vi "Actor Core.vi"(8 "error in":errorcluster, 11 "SLM_Controller in":refnum<class "SLM_Controller.lvclass">) -> (0 "error out":errorcluster, 3 "Actor out":refnum<class "Actor.lvclass">)   [LabVIEW 2023, in "SLM_Controller.lvlib" / "SLM_Controller.lvclass"]
doc: "(<B>Filename</B>: Actor Framework.lvlib:Actor.lvclass:Actor Core.vi)\n\nReceives messages to the actor, reacts to them, and initiates any error handling that may shut the actor down.\n\nDescendant classes may override this VI to append parallel tasks for the actor to complete while it handles messages. Overrides use the Call Parent Class Method node."
uses:
  SLM_Controller.lvclass
  C:/Program Files/National Instruments/LabVIEW 2023/vi.lib/ActorFramework/Actor/Actor.lvclass
  <vilib>/ActorFramework/Actor/Actor.lvclass
  <vilib>/ActorFramework/Actor/Actor.lvclass/Actor.ctl
  <vilib>/ActorFramework/Message Enqueuer/Message Enqueuer.lvclass/Message Enqueuer.ctl
  <vilib>/ActorFramework/Message Enqueuer/Init from Existing Queue.vi
  <vilib>/ActorFramework/Message Enqueuer/Enqueue.vi
  <vilib>/ActorFramework/Stop Msg/Stop Msg.lvclass
  C:/Program Files/National Instruments/LabVIEW 2023/vi.lib/ActorFramework/Message/Message.lvclass
  <vilib>/ActorFramework/Message Priority Queue/Priority Enqueue.vi
  <vilib>/ActorFramework/Message Enqueuer/Message Enqueuer.lvclass
  SLM_Controller.lvclass/SLM_Controller.ctl
panel:
  out "Main Control Path":path
  out "function name out":errorcluster
  out "Python Session":refnum<k35>
  out "Python Scripts Path":path
  out "VI":refnum<vi>
  out "Phase Array Graph":dbl[][](graph)
  in  "Continuous Button":bool
  in  "Correction Pattern":path=path "C:/Users/quantum/Documents/LVDAQ/ConcreteClasses/ConcreteInstrumentClasses/SLMClasses/Hamamatsu_X13138/Resources/correction_pattern_13138/CAL_LSH0802650_810nm.bmp"
  in  "SLM Monitor":i32=2
  in  "Modulation Depth":dbl=214.0
  in  "Initialize SLM":bool
  in  "Grating Sliders":cluster{"Y":sgl, "X":sgl} {"X" min=0 max=10 step=0.01 scale=0.0..10.0; "Y" min=0 max=10 step=0.01 scale=0.0..10.0}
  out "SLM Final Phase":dbl[][](graph)
  in  "Single Upload":bool
  in  "SLM Size":i32=800
  in  "Phase Array":dbl[][](array[numeric])
  in  "MegaPixels Y":i32=4
  in  "MegaPixels X":i32=4
  in  "Start/Stop":bool
  in  "Phase Scan ON / OFF":bool
  in  "Phase Scan":u16(ring) items=["2x1", "1x2", "2x2"]
  # "X"
  # "Y"
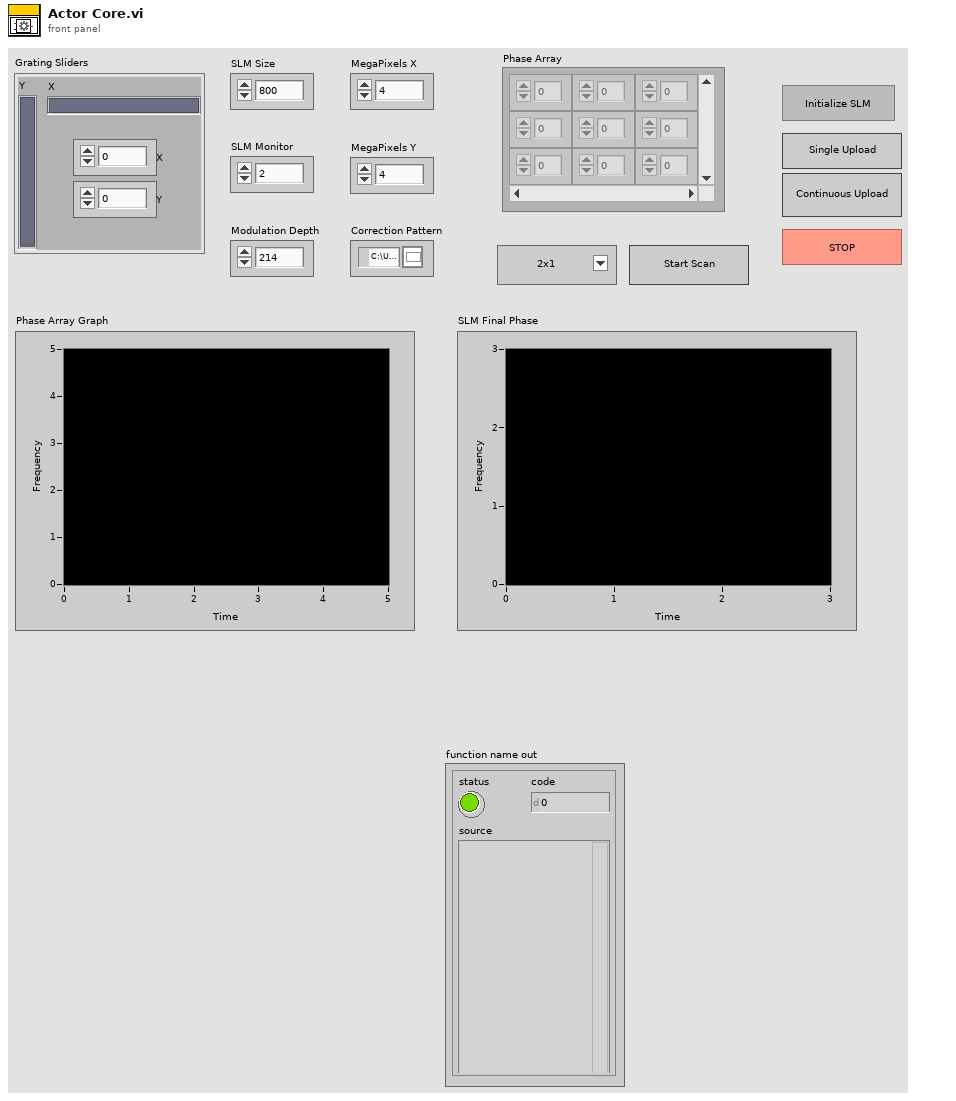
[diagram p1: front panel]
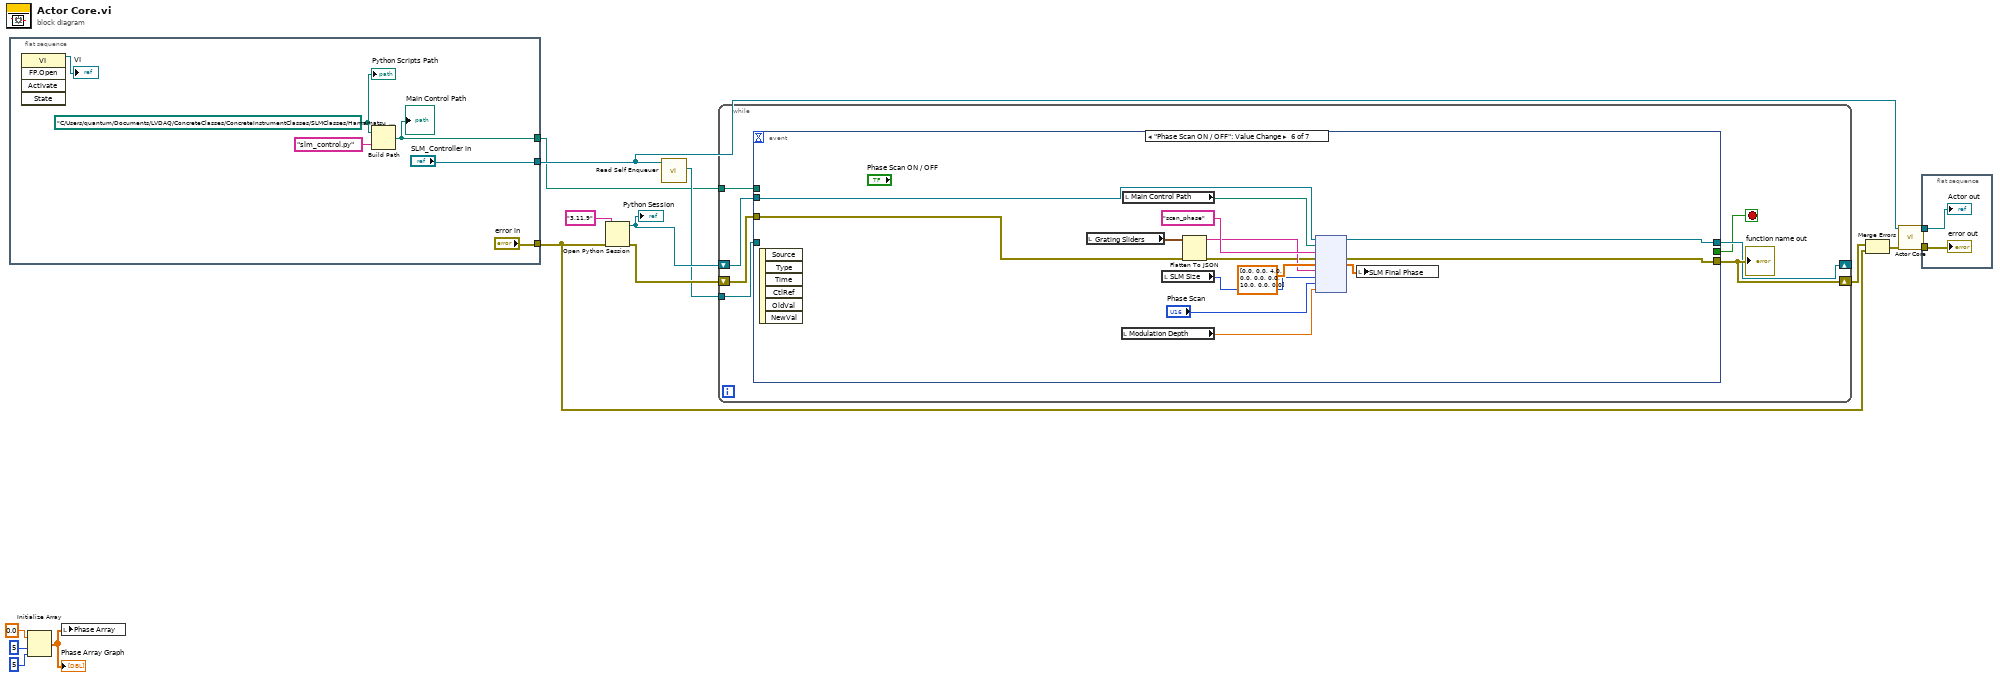
[diagram p0: block diagram]
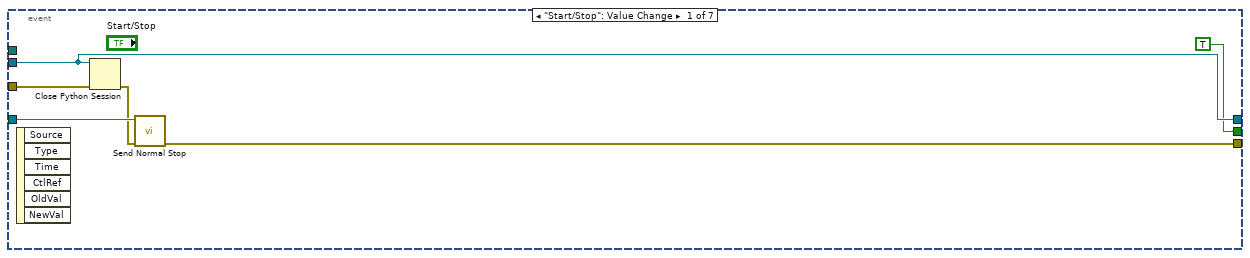
[diagram p2: hidden frame]
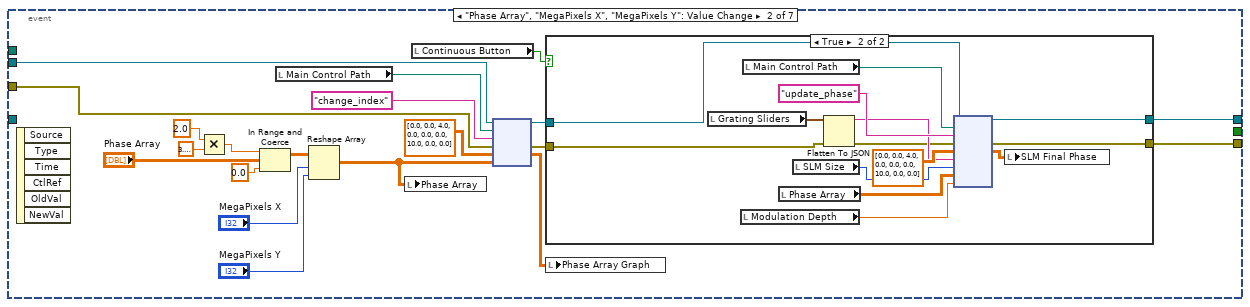
[diagram p3: hidden frame]
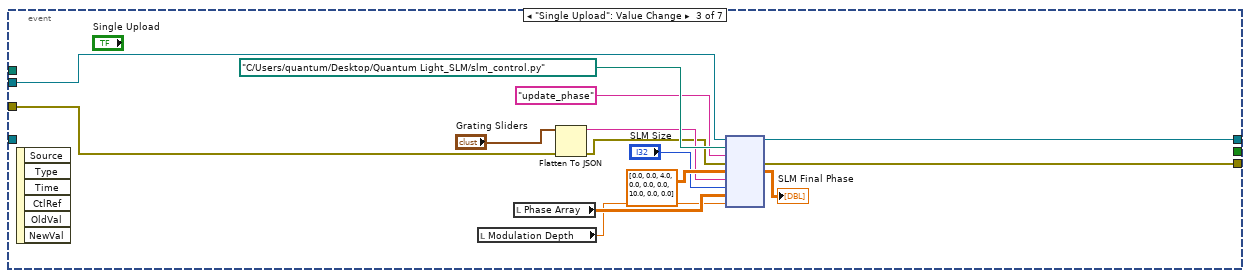
[diagram p5: hidden frame]
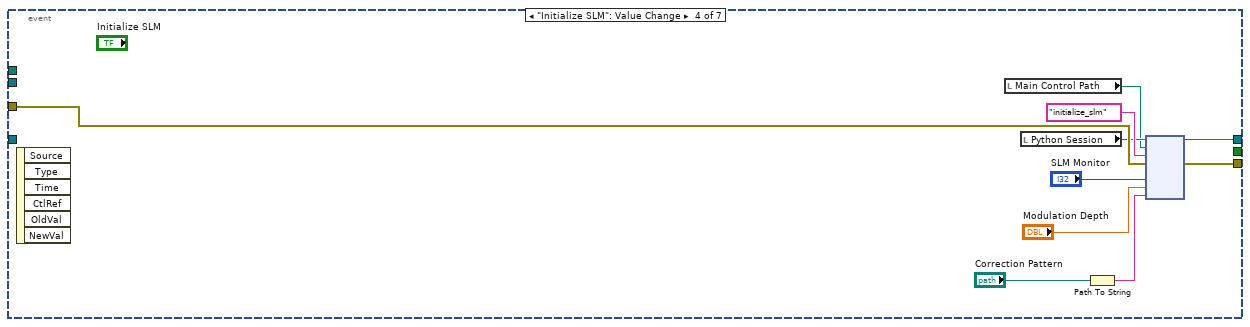
[diagram p6: hidden frame]
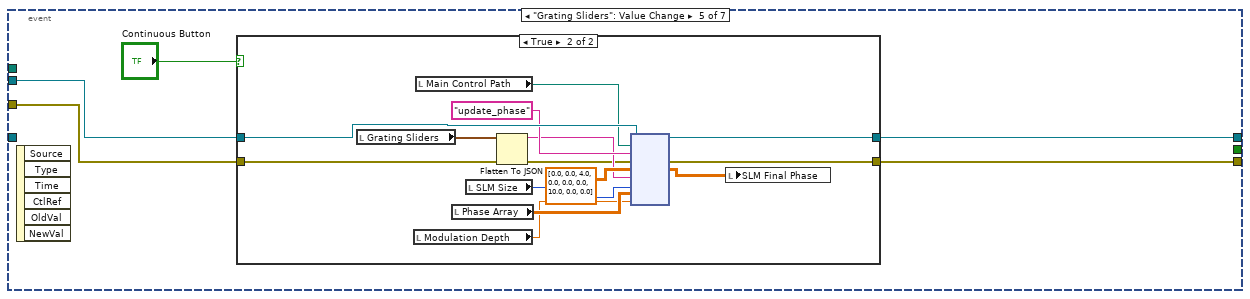
[diagram p7: hidden frame]
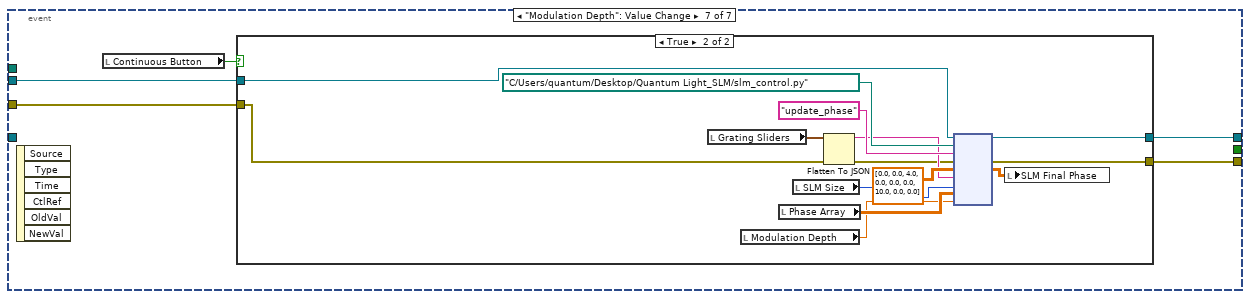
[diagram p9: hidden frame]
diagram:
  n1 = flat-sequence {
    tunnel: ["error in"] -> w7
    tunnel: ["SLM_Controller in"] -> w6
    tunnel: [w16] -> w1
    frame #0 {
      w17 = path "C:/Users/quantum/Documents/LVDAQ/ConcreteClasses/ConcreteInstrumentClasses/SLMClasses/Hamamatsu_X13138/Resources/Python" ("module path")
      n2 = invoke class="VI" method="FP.Open"() -> (reference out=→"VI":refnum<vi>)  [unwired: 5 in, 4 out]
      n3 = Build Path(base path=w17, name or relative path="slm_control.py") -> (appended path=w16:path)
      "Main Control Path" <- w16
      "Python Scripts Path" <- w17
    }
  }
  n4 = Initialize Array(0.0 ("element"), 5 ("dimension size"), 5 ("dimension size")) -> (w9:dbl[][])
  "Phase Array Graph" <- w9
  n5 = local write "Phase Array"(w9) -> ()
  n6 = Open Python Session(python version="3.11.9" ("Python version"), 3:w7) -> (session out=w15:refnum<k35>, error out=w14:errorcluster)  [unwired: 1 in]
  "Python Session" <- w15
  n7 = call <vilib>:"Read Self Enqueuer.vi"("Actor"=w6) -> ("Self Enqueuer"=w5:refnum<class "Message Enqueuer.lvclass">)  [unwired: 10 in]
  n8 = while {
    shift-right: [w25] -> _
    shift-left: w15 -> [w28]
    shift-right: [w26] -> w8
    shift-left: w14 -> [w27]
    tunnel: w5 -> [w23]
    tunnel: w1 -> [w22]
    stop <- w24 stop-if-true
    n9 = event shown="[5] \"Phase Scan ON / OFF\": Value Change" {
      selector: _ -> [_ _ _ _ _ _ _]
      dyn-events: _ -> [_ _ _ _ _ _ _]
      timeout: _ -> [_ _ _ _ _ _ _]
      tunnel: w28 -> [w33 w48 w84 _ w99 w129 w134]
      tunnel: w27 -> [w34 w47 w73 w94 w98 w128 w133]
      tunnel: [w29 w38 w82 w92 w96 w126 w131] -> w26
      tunnel: [w33 w39 w83 w93 w97 w127 w132] -> w25
      tunnel: [TRUE ("Start/Stop") _ _ _ _ _ _] -> w24
      tunnel: w23 -> [w31 _ _ _ _ _ _]
      tunnel: w22 -> [_ _ _ _ _ _ _]
      event "Start/Stop": Value Change {
        n10 = event-data() -> ()  [unwired: 1 in, 6 out]
        n11 = Close Python Session(session in=w33, error in=w34) -> (11:w30:errorcluster)
        n12 = call <vilib>:"Send Normal Stop.vi"("error in (no error)"=w30, "Message Enqueuer"=w31) -> ("error out"=w29:errorcluster)  [unwired: 9 in]
      }
      event "Phase Array", "MegaPixels X", "MegaPixels Y": Value Change {
        n13 = event-data() -> ()  [unwired: 1 in, 6 out]
        n14 = Multiply(x=2.0, y=3.141592653589793) -> (x*y=w52:dbl)
        n15 = In Range and Coerce(upper limit=w52, x="Phase Array", lower limit=0.0) -> (coerced(x)=w53:dbl[][])  [unwired: 1 out]
        n16 = local read "Main Control Path"() -> (w35:path)
        n17 = Reshape Array "Reshape Array"(w53, "MegaPixels X", "MegaPixels Y") -> (w36:dbl[][])
        n18 = local write "Phase Array"(w36) -> ()
        n19 = local read "Continuous Button"() -> (w40:bool)
        n20 = node(w48, w35, "change_index" ("function name"), w47, dbl[][] [[0.0, 0.0, 4.0], [0.0, 0.0, 0.0], [10.0, 0.0, 0.0]] ("Python Graph"), w36) -> (w41:refnum<k35>, w42:errorcluster, w37:dbl[][])  [unwired: 1 in, 2 out]
        n21 = case shown="True" w40 {
          tunnel: w41 -> [w55 w70]
          tunnel: w42 -> [w56 w61]
          tunnel: [w55 w69] -> w39
          tunnel: [w56 w68] -> w38
          frame False {
          }
          frame True {
            n22 = local read "Grating Sliders"() -> (w63:cluster{"Y":sgl, "X":sgl})
            n23 = local read "Modulation Depth"() -> (w59:dbl)
            n24 = local read "Main Control Path"() -> (w57:path)
            n25 = local read "Phase Array"() -> (w58:dbl[][])
            n26 = local read "SLM Size"() -> (w64:i32)
            n27 = Flatten To JSON(anything=w63, error in (no error)=w61) -> (JSON string=w62:string, 11:w60:errorcluster)  [unwired: 1 in]
            n28 = node(w70, w57, "update_phase" ("function name"), w60, dbl[][] [[0.0, 0.0, 4.0], [0.0, 0.0, 0.0], [10.0, 0.0, 0.0]] ("Python Graph"), w62, w64, w58, w59) -> (w69:refnum<k35>, w68:errorcluster, w65:dbl[][])  [unwired: 4 in, 2 out]
            n29 = local write "SLM Final Phase"(w65) -> ()
          }
        }
        n30 = local write "Phase Array Graph"(w37) -> ()
      }
      event "Single Upload": Value Change {
        n31 = event-data() -> ()  [unwired: 1 in, 6 out]
        n32 = local read "Modulation Depth"() -> (w71:dbl)
        n33 = local read "Phase Array"() -> (w77:dbl[][])
        n34 = Flatten To JSON(anything="Grating Sliders", error in (no error)=w73) -> (JSON string=w74:string, 11:w72:errorcluster)  [unwired: 1 in]
        n35 = node(w84, path "C:/Users/quantum/Desktop/Quantum Light_SLM/slm_control.py" ("module path"), "update_phase" ("function name"), w72, dbl[][] [[0.0, 0.0, 4.0], [0.0, 0.0, 0.0], [10.0, 0.0, 0.0]] ("Python Graph"), w74, "SLM Size", w77, w71) -> (w83:refnum<k35>, w82:errorcluster, →"SLM Final Phase":dbl[][])  [unwired: 4 in, 2 out]
      }
      event "Initialize SLM": Value Change {
        n36 = event-data() -> ()  [unwired: 1 in, 6 out]
        n37 = local read "Main Control Path"() -> (w85:path)
        n38 = local read "Python Session"() -> (w86:refnum<k35>)
        n39 = Path To String(path="Correction Pattern") -> (string=w88:string)
        n40 = node(w86, w85, "initialize_slm" ("function name"), w94, "SLM Monitor", "Modulation Depth", w88) -> (w93:refnum<k35>, w92:errorcluster)  [unwired: 5 in, 2 out]
      }
      event "Grating Sliders": Value Change {
        n41 = event-data() -> ()  [unwired: 1 in, 6 out]
        n42 = case shown="True" "Continuous Button" {
          tunnel: w99 -> [w100 w115]
          tunnel: w98 -> [w101 w105]
          tunnel: [w100 w114] -> w97
          tunnel: [w101 w113] -> w96
          frame False {
          }
          frame True {
            n43 = local read "Grating Sliders"() -> (w107:cluster{"Y":sgl, "X":sgl})
            n44 = local read "Modulation Depth"() -> (w103:dbl)
            n45 = local read "Main Control Path"() -> (w102:path)
            n46 = local read "Phase Array"() -> (w109:dbl[][])
            n47 = local read "SLM Size"() -> (w108:i32)
            n48 = Flatten To JSON(anything=w107, error in (no error)=w105) -> (JSON string=w106:string, 11:w104:errorcluster)  [unwired: 1 in]
            n49 = node(w115, w102, "update_phase" ("function name"), w104, dbl[][] [[0.0, 0.0, 4.0], [0.0, 0.0, 0.0], [10.0, 0.0, 0.0]] ("Python Graph"), w106, w108, w109, w103) -> (w114:refnum<k35>, w113:errorcluster, w110:dbl[][])  [unwired: 4 in, 2 out]
            n50 = local write "SLM Final Phase"(w110) -> ()
          }
        }
      }
      event "Phase Scan ON / OFF": Value Change {
        n51 = event-data() -> ()  [unwired: 1 in, 6 out]
        n52 = local read "Grating Sliders"() -> (w121:cluster{"Y":sgl, "X":sgl})
        n53 = local read "Modulation Depth"() -> (w118:dbl)
        n54 = local read "Main Control Path"() -> (w117:path)
        n55 = local read "SLM Size"() -> (w122:i32)
        n56 = Flatten To JSON(anything=w121, error in (no error)=w128) -> (JSON string=w120:string, 11:w119:errorcluster)  [unwired: 1 in]
        n57 = node(w129, w117, "scan_phase" ("function name"), w119, dbl[][] [[0.0, 0.0, 4.0], [0.0, 0.0, 0.0], [10.0, 0.0, 0.0]] ("Python Graph"), w120, w122, "Phase Scan", w118) -> (w127:refnum<k35>, w126:errorcluster, w123:dbl[][])  [unwired: 4 in, 2 out]
        n58 = local write "SLM Final Phase"(w123) -> ()
      }
      event "Modulation Depth": Value Change {
        n59 = event-data() -> ()  [unwired: 1 in, 6 out]
        n60 = local read "Continuous Button"() -> (w130:bool)
        n61 = case shown="True" w130 {
          tunnel: w134 -> [w135 w150]
          tunnel: w133 -> [w136 w139]
          tunnel: [w135 w149] -> w132
          tunnel: [w136 w148] -> w131
          frame False {
          }
          frame True {
            n62 = local read "Grating Sliders"() -> (w141:cluster{"Y":sgl, "X":sgl})
            n63 = local read "Modulation Depth"() -> (w137:dbl)
            n64 = local read "Phase Array"() -> (w143:dbl[][])
            n65 = local read "SLM Size"() -> (w142:i32)
            n66 = Flatten To JSON(anything=w141, error in (no error)=w139) -> (JSON string=w140:string, 11:w138:errorcluster)  [unwired: 1 in]
            n67 = node(w150, path "C:/Users/quantum/Desktop/Quantum Light_SLM/slm_control.py" ("module path"), "update_phase" ("function name"), w138, dbl[][] [[0.0, 0.0, 4.0], [0.0, 0.0, 0.0], [10.0, 0.0, 0.0]] ("Python Graph"), w140, w142, w143, w137) -> (w149:refnum<k35>, w148:errorcluster, w144:dbl[][])  [unwired: 4 in, 2 out]
            n68 = local write "SLM Final Phase"(w144) -> ()
          }
        }
      }
    }
    "function name out" <- w26
  }
  n69 = Merge Errors(w8, w7) -> (w4:errorcluster)
  n70 = call-parent "Actor Core.vi"("error in"=w4, "Actor in"=w6) -> ("error out"=w3:errorcluster, "Actor out"=w2:refnum<class "Actor.lvclass">)  [unwired: 8 in]
  n71 = flat-sequence {
    tunnel: w3 -> [w152]
    tunnel: w2 -> [w151]
    frame #0 {
      "error out" <- w152
      "Actor out" <- w151
    }
  }
